vi "report_write_go.vi"   [LabVIEW 2014]
uses:
  g_ReportControl.vi
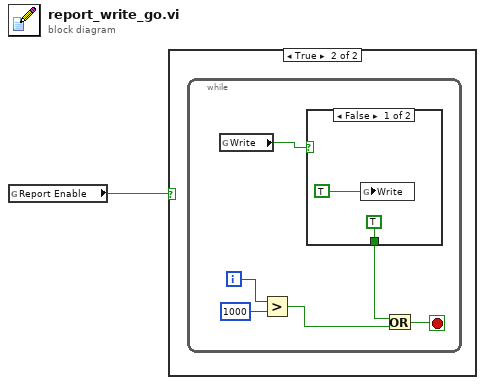
[diagram p0: block diagram]
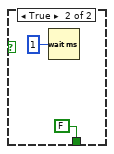
[diagram p3: hidden frame]
diagram:
  n1 = global read "g_ReportControl.vi" "Report Enable"() -> (w1:bool)
  n2 = case shown="True" w1 {
    frame False {
    }
    frame True {
      n3 = while {
        i -> [w2]
        stop <- w5 stop-if-true
        n4 = global read "g_ReportControl.vi" "Write"() -> (w7:bool)
        n5 = Greater?(x=w2, y=1000) -> (0:w3:bool)
        n6 = case shown="False" w7 {
          tunnel: [TRUE FALSE] -> w4
          frame False {
            n7 = global write "g_ReportControl.vi" "Write"(TRUE ("Send")) -> ()
          }
          frame True {
            n8 = Wait (ms)(milliseconds to wait=u32 1) -> ()  [unwired: 1 out]
          }
        }
        n9 = Or(x=w4, y=w3) -> (x .or. y?=w5:bool)
      }
    }
  }
